vi "CloseScanFile.vi"(8 "error in":errorcluster, 11 "refnum":refnum<file>) -> (0 "error out":errorcluster)   [LabVIEW 2012]
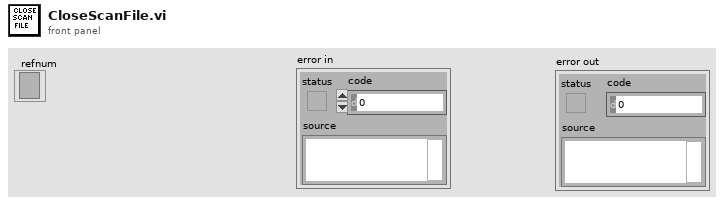
[diagram p1: front panel]
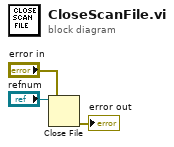
[diagram p0: block diagram]
diagram:
  n1 = Close File(refnum="refnum", error in="error in") -> (error out=→"error out":errorcluster)  [unwired: 1 out]
